vi "Loop_SEN_Limit.vi"() -> ()   [LabVIEW 2017, in "Claw.lvlib"]
uses:
  Claw.lvlib
  CLUSTER_Limit_Switch_Output.ctl
  Globals/Global_Device_IDs.vi
  <vilib>/Rock Robotics/WPI/Switch/WPI_SwitchOpenLimit.vi
  _SHARE ALL/Global Share All/Global_STOP.vi
  Global_ACT Write_Data Out.vi
panel:
  out "Limit Switch Output":T1
  out "Cycle Time (S)":dbl format="%.3g"
  in  "Target Time(ms)":u32=50
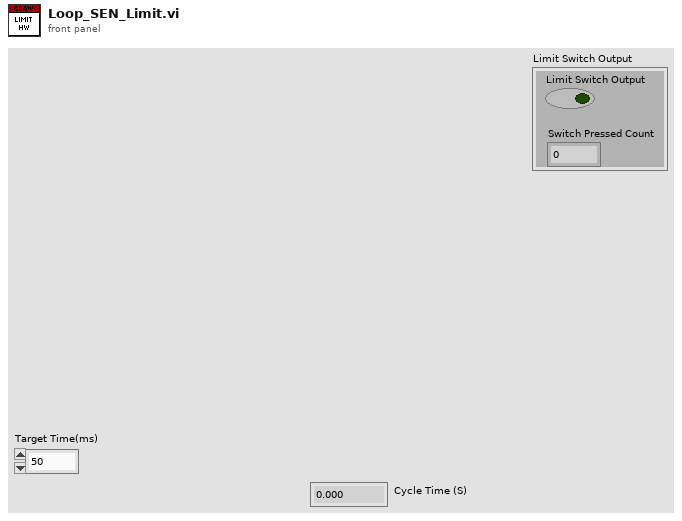
[diagram p1: front panel]
types:
  T1 = typedef "Claw.lvlib/CLUSTER_Limit_Switch_Output.ctl" = cluster{"Limit Switch Output":bool, "Switch Pressed Count":i32}
  T2 = typedef "CLUSTER_Claw_Setup.ctl" = cluster{"Left Motor Setup":T3, "Right Motor Setup":T3, "Left Motor PDP":i32, "Right Motor PDP":i32, "Solonoid Setup":T5, "Limit Switch DIO":T7}
  T3 = typedef "CLUSTER_PWM Motor Setup.ctl" = cluster{"Motor PWM":T4, "Invert Motor":bool}
  T4 = typedef "FPGA_DIOPWMChannel.ctl" = enum8{"PWM 0", "PWM 1", "PWM 2", "PWM 3", "PWM 4", "PWM 5", "PWM 6", "PWM 7", "PWM 8", "PWM 9", "PWM MXP 0", "PWM MXP 1", "PWM MXP 2", "PWM MXP 3", "PWM MXP 4", "PWM MXP 5", "PWM MXP 6", "PWM MXP 7", "PWM MXP 8", "PWM MXP 9", "Invalid"}
  T5 = typedef "CLUSTER_Solonoid_Setup.ctl" = cluster{"Pneumatics Control Module (0)":u8, "Forward Solenoid Channel":T6, "Reverse Solenoid Channel":T6}
  T6 = typedef "WPI_SolenoidChannel.ctl" = enum8{"Solenoid 0", "Solenoid 1", "Solenoid 2", "Solenoid 3", "Solenoid 4", "Solenoid 5", "Solenoid 6", "Solenoid 7", "Invalid"}
  T7 = typedef "FPGA_DIOChannel.ctl" = enum8{"DIO 0", "DIO 1", "DIO 2", "DIO 3", "DIO 4", "DIO 5", "DIO 6", "DIO 7", "DIO 8", "DIO 9", "DIO MXP 0", "DIO MXP 1", "DIO MXP 2", "DIO MXP 3", "DIO MXP 4", "DIO MXP 5", "DIO MXP 6", "DIO MXP 7", "DIO MXP 8", "DIO MXP 9", "DIO MXP 10", "DIO MXP 11", "DIO MXP 12", "DIO MXP 13", "DIO MXP 14", "DIO MXP 15", "SPI Port CS1", "SPI Port CS2", "SPI Port CS3", "SPI Port MISO", "SPI Port MOSI", "Invalid"}
  T8 = typedef "WPI_SwitchDevRef.ctl" = cluster{"DevStatus":errorcluster, "DIO Channel":T7, "CntIndex":T9, "Normally Closed":bool}
  T9 = typedef "FPGA_CounterCtrSystemIndex.ctl" = enum8{"Ctr 0", "Ctr 1", "Ctr 2", "Ctr 3", "Ctr 4", "Ctr 5", "Ctr 6", "Ctr 7", "Invalid"}
  T10 = cluster{"SwitchDevRef":T8, "Limit Switch Output":T1, "Target Time(ms)":u32, "Current Time":timestamp, "Previous Time":timestamp, "Cycle Time (S)":dbl}
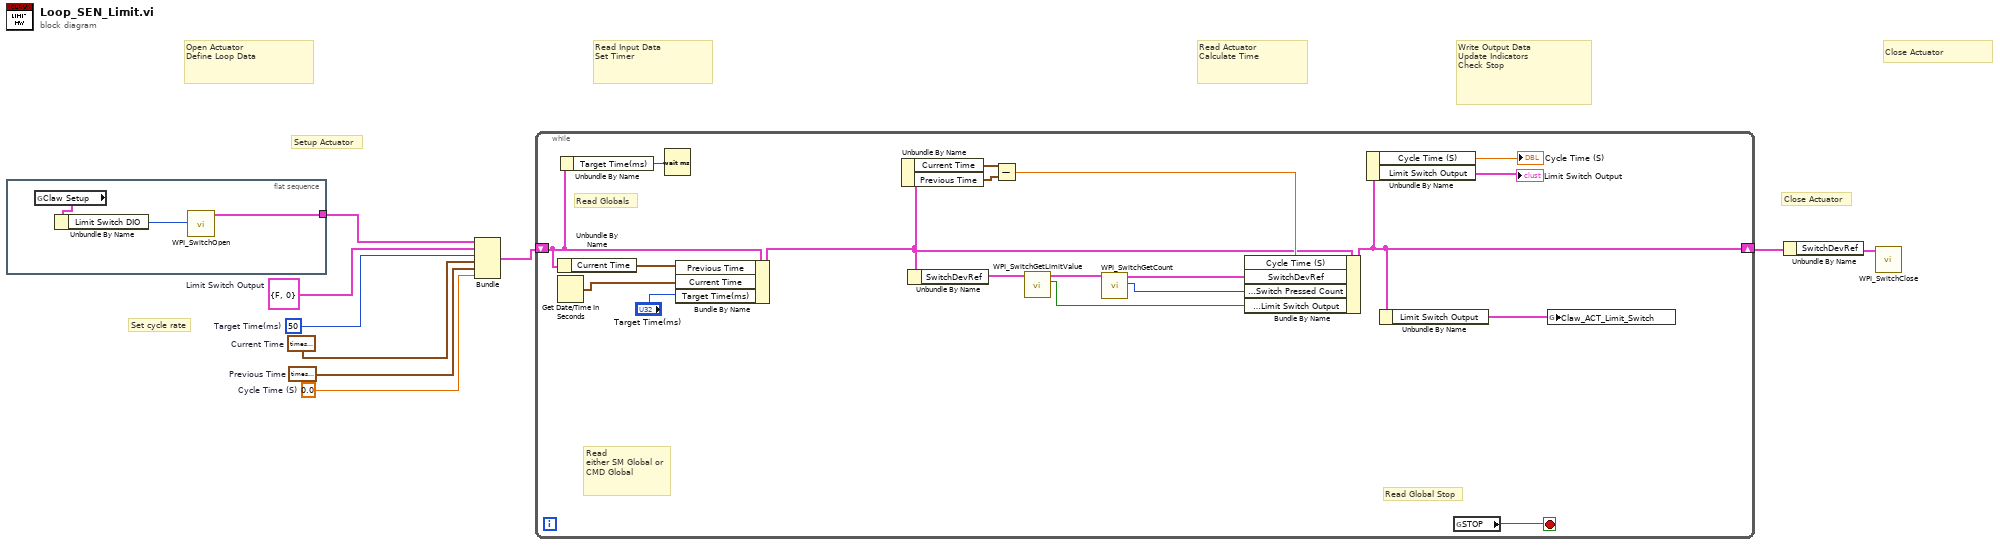
[diagram p0: block diagram]
diagram:
  w2 = T1 {"Limit Switch Output"=FALSE, "Switch Pressed Count"=0}  # Limit Switch Output
  w4 = 0.0  # Cycle Time (S)
  w9 = timestamp(0 s since 1904-01-01)  # Previous Time
  w8 = timestamp(0 s since 1904-01-01)  # Current Time
  w7 = u32 50  # Target Time(ms)
  # "Close Actuator"
  # "Write Output Data\nUpdate Indicators\nCheck Stop"
  # "Read Actuator\nCalculate Time"
  # "Read Input Data\nSet Timer"
  # "Open Actuator\nDefine Loop Data"
  # "Set cycle rate"
  # "Close Actuator"
  # "Setup Actuator"
  n1 = flat-sequence {
    tunnel: [w11] -> w3
    frame #0 {
      n2 = global read "Global_Device_IDs.vi" "Claw Setup"() -> (w12:T2)
      n3 = Unbundle By Name(w12) -> ("Limit Switch DIO"=w10:T7)
      n4 = call-poly <vilib>:"WPI_SwitchOpen.vi"("DIO Channel"=w10) -> ("SwitchDevRef"=w11:T8)  [unwired: 9 in, 1 out]
    }
  }
  n5 = Bundle("SwitchDevRef"=w3, "Limit Switch Output"=w2, "Target Time(ms)"=w7, "Current Time"=w8, "Previous Time"=w9, "Cycle Time (S)"=w4) -> (w6:T10)  [unwired: 1 in]
  n6 = while {
    shift-right: [w23] -> w5
    shift-left: w6 -> [w25]
    stop <- w31 stop-if-true
    # "Read\neither SM Global or CMD Global"
    # "Read Globals"
    # "Read Global Stop"
    n7 = Unbundle By Name(w25) -> ("Current Time"=w29:timestamp)
    n8 = Get Date/Time In Seconds() -> (seconds since 1Jan1904=w30:timestamp)
    n9 = Unbundle By Name(w25) -> ("Target Time(ms)"=w24:u32)
    n10 = Wait (ms)(milliseconds to wait=w24) -> ()  [unwired: 1 out]
    n11 = Bundle By Name(cluster=w25, "Previous Time"=w29, "Current Time"=w30, "Target Time(ms)"="Target Time(ms)") -> (w20:T10)
    n12 = Unbundle By Name(w20) -> ("Current Time"=w28:timestamp, "Previous Time"=w27:timestamp)
    n13 = Unbundle By Name(w20) -> ("SwitchDevRef"=w18:T8)
    n14 = Subtract(x=w28, y=w27) -> (x-y=w21:dbl)
    n15 = call <vilib>:"WPI_SwitchGetLimitValue.vi"("SwitchDevRef"=w18) -> ("Switch Pressed"=w14:bool, "SwitchDevRef"=w17:T8)  [unwired: 8 in, 1 out]
    n16 = call <vilib>:"WPI_SwitchGetCount.vi"("SwitchDevRef"=w17) -> ("Switch Pressed Count"=w15:i32, "SwitchDevRef"=w16:T8)  [unwired: 8 in, 1 out]
    n17 = Bundle By Name(cluster=w20, "Cycle Time (S)"=w21, "SwitchDevRef"=w16, "Limit Switch Output.Switch Pressed Count"=w15, "Limit Switch Output.Limit Switch Output"=w14) -> (w23:T10)
    n18 = Unbundle By Name(w23) -> ("Cycle Time (S)"=→"Cycle Time (S)":dbl, "Limit Switch Output"=→"Limit Switch Output":T1)
    n19 = Unbundle By Name(w23) -> ("Limit Switch Output"=w19:T1)
    n20 = global read "Global_STOP.vi" "STOP"() -> (w31:bool)
    n21 = global write "Global_ACT Write_Data Out.vi" "Claw_ACT_Limit_Switch"(w19) -> ()
  }
  n22 = Unbundle By Name(w5) -> ("SwitchDevRef"=w1:T8)
  n23 = call <vilib>:"WPI_SwitchClose.vi"("SwitchDevRef"=w1) -> ()  [unwired: 10 in, 1 out]
